vi "Ms_to_samples.vi"(6 "Sampling rate (Hz)":dbl, 11 "Step duration (ms)":dbl) -> (3 "Numeric":i32)   [LabVIEW 2016]
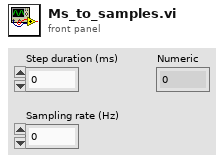
[diagram p1: front panel]
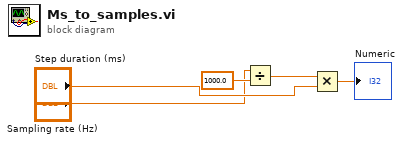
[diagram p0: block diagram]
diagram:
  n1 = Divide(x="Sampling rate (Hz)", y=1000.0) -> (x/y=w3:dbl)
  n2 = Multiply(x=w3, y="Step duration (ms)") -> (x*y=→"Numeric":dbl)
